vi "Format To Doller String.vi"() -> ()   [LabVIEW 2019]
panel:
  out "String 2":string
  out "error":string
  in  "String":string
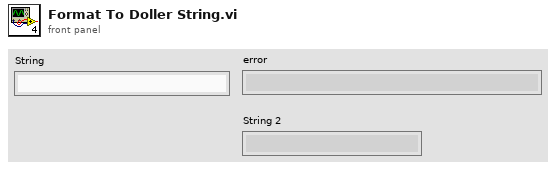
[diagram p1: front panel]
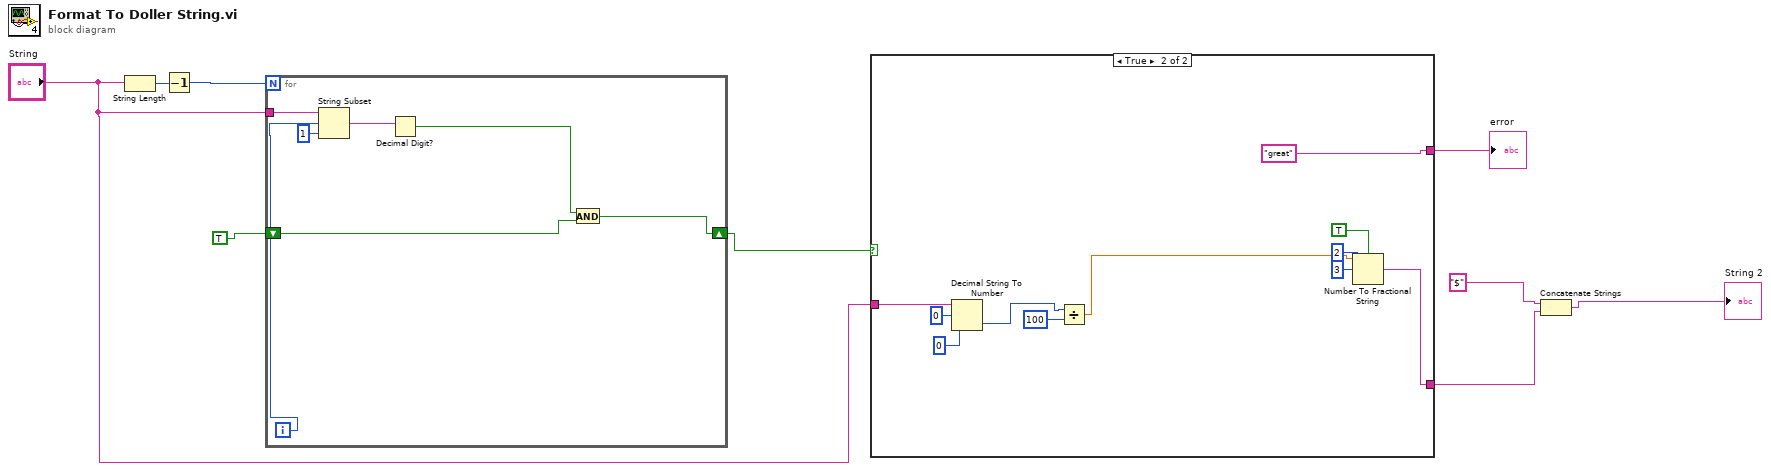
[diagram p0: block diagram]
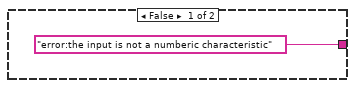
[diagram p2: hidden frame]
diagram:
  n1 = String Length(string="String") -> (length=w9:i32)
  n2 = Decrement(x=w9) -> (x-1=w5:i32)
  n3 = for {
    N: w5 -> [_]
    tunnel: "String" -> [w16]
    shift-right: [w11] -> w8
    shift-left: TRUE -> [w12]
    i -> [w15]
    n4 = String Subset(string=w16, offset (0)=w15, length (rest)=1 ("length (rest)")) -> (substring=w13:string)
    n5 = Decimal Digit?(1:w13) -> (0:w10:bool)
    n6 = And(x=w10, y=w12) -> (x .and. y?=w11:bool)
  }
  n7 = case shown="True" w8 {
    tunnel: ["error:the input is not a numberic characteristic" "great"] -> w6
    tunnel: "String" -> [_ w27]
    tunnel: [_ w19] -> w1
    frame False {
    }
    frame True {
      n8 = Decimal String To Number(string=w27, offset=0, default (0L)=0 ("default (0 I32)")) -> (number=w23:i32)  [unwired: 1 out]
      n9 = Divide(x=w23, y=100) -> (x/y=w21:dbl)
      n10 = Number To Fractional String(use system decimal point (T)=TRUE, number=w21, width (-)=i16 3, precision (6)=i16 2) -> (F-format string=w19:string)
    }
  }
  "error" <- w6
  n11 = Concatenate Strings("$", w1) -> (→"String 2":string)
